vi "Enqueue Message.vi"(8 "error in (no error)":errorcluster, 9 "Message Priority (Normal)":T1=enum."Normal", 10 "Message":refnum<class "Message.lvclass">, 11 "Interlock Q Class in":refnum<class "Interlock Q Class.lvclass">) -> (0 "error out":errorcluster, 3 "Interlock Q Class out":refnum<class "Interlock Q Class.lvclass">)   [LabVIEW 2022 SP3, in "Interlock Q Class.lvclass"]
uses:
  Interlock Q Class.lvclass
  <vilib>/ActorFramework/Message Enqueuer/Message Priority.ctl
  <vilib>/ActorFramework/Message/Message.lvclass
  Interlock Q Class.lvclass/Interlock Q Class.ctl
  Process State Data/Process State Data.lvclass/Process State Data.ctl
  <vilib>/ActorFramework/Message Enqueuer/Message Enqueuer.lvclass/Message Enqueuer.ctl
  Process State Data/Accessor/Write Busy.vi
  Process State Data/Accessor/Write Proccess Error.vi
  Process State Data/Accessor/Read Busy.vi
  <vilib>/ActorFramework/Message Priority Queue/Priority Enqueue.vi
  <vilib>/Utility/error.llb/Error Cluster From Error Code.vi
  <vilib>/ErrorRing/Error Ring.xnode
  <vilib>/ActorFramework/Message Enqueuer/Message Enqueuer.lvclass
  Process State Data/Process State Data.lvclass
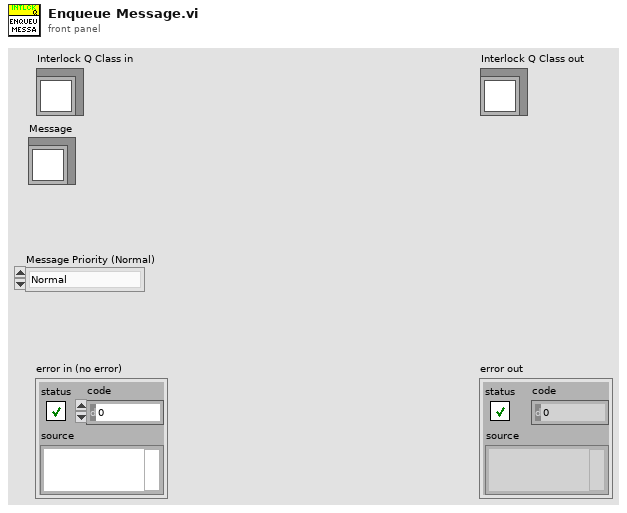
[diagram p1: front panel]
types:
  T1 = typedef "Actor Framework.lvlib/Message Enqueuer.lvclass/Message Priority.ctl" = enum16{"Low", "Normal", "High"}
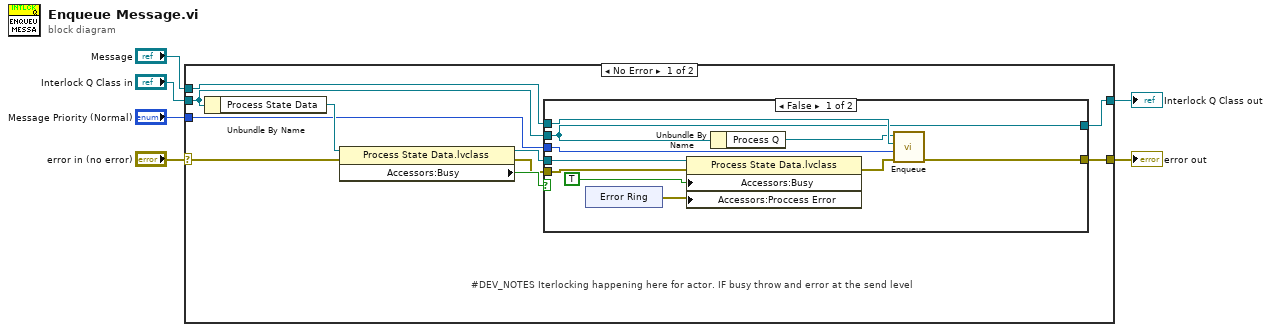
[diagram p0: block diagram]
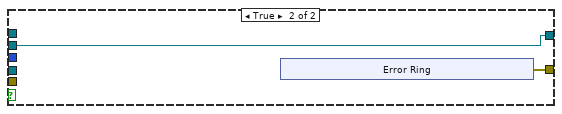
[diagram p2: hidden frame]
diagram:
  n1 = case shown="No Error" "error in (no error)" {
    selector: "error in (no error)" -> [w9 w36]
    tunnel: [w13 w36] -> w5
    tunnel: [w7 w35] -> w3
    tunnel: "Interlock Q Class in" -> [w8 w35]
    tunnel: "Message" -> [w15 _]
    tunnel: "Message Priority (Normal)" -> [w14 _]
    frame No Error {
      # "#DEV_NOTES Iterlocking happening here for actor. IF busy throw and error at the send level"
      n2 = Unbundle By Name(w8) -> ("Process State Data"=w16:refnum<data-value>)
      n3 = property class="Process State Data.lvclass"(reference=w16, error in=w9) -> (reference out=w11:refnum<data-value>, error out=w10:errorcluster, "Accessors:Busy"=w12:bool)
      n4 = case shown="False" w12 {
        tunnel: w15 -> [w26 _]
        tunnel: w14 -> [w25 _]
        tunnel: [w24 w29] -> w13
        tunnel: w11 -> [w23 _]
        tunnel: w10 -> [w21 _]
        tunnel: w8 -> [w18 w28]
        tunnel: [w18 w28] -> w7
        frame False {
          n5 = xnode "Error Ring"() -> ("error out"=w17:errorcluster)
          n6 = property class="Process State Data.lvclass"(reference=w23, error in=w21, "Accessors:Busy"=TRUE ("Busy"), "Accessors:Proccess Error"=w17) -> (error out=w20:errorcluster)  [unwired: 1 out]
          n7 = Unbundle By Name(w18) -> ("Process Q"=w19:refnum<class "Message Enqueuer.lvclass">)
          n8 = call <vilib>:"Enqueue.vi"("error in (no error)"=w20, "Message Priority (Normal)"=w25, "Message"=w26, "Message Enqueuer in"=w19) -> ("error out"=w24:errorcluster)  [unwired: 6 in, 1 out]
        }
        frame True {
          n9 = xnode "Error Ring"() -> ("error out"=w29:errorcluster)
        }
      }
    }
    frame Error {
    }
  }
  "error out" <- w5
  "Interlock Q Class out" <- w3
